vi "Can Rock Fall Down.vi"(0 "Position in Chamber to Check":i32, 1 "Chamber":u32[][](array[colorbox]), 2 "Rock":u32[][](array[colorbox])) -> (3 "Can Rock Fall Down ?":bool=TRUE)   [LabVIEW 2020, in "AoC 2022.lvlib"]
uses:
  AoC 2022.lvlib
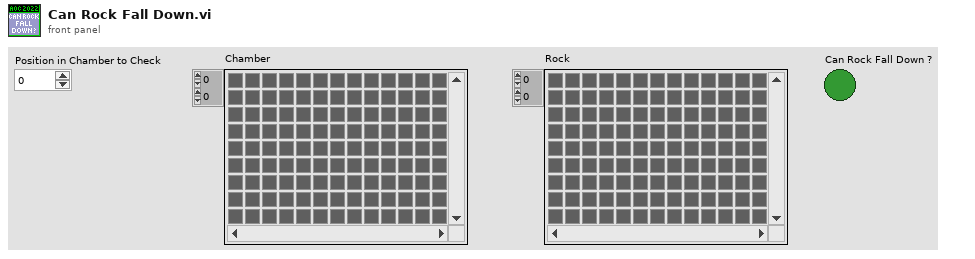
[diagram p1: front panel]
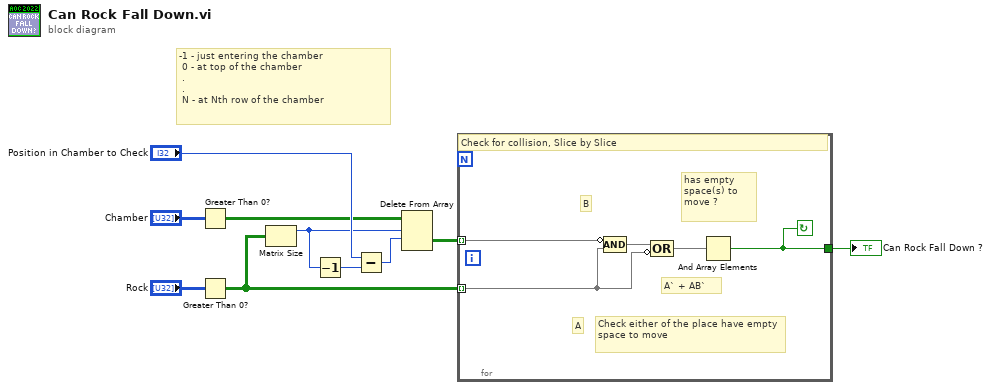
[diagram p0: block diagram]
diagram:
  # "-1 - just entering the chamber\n 0 - at top of the chamber\n .\n .\n N - at Nth row of the chamber"
  n1 = Greater Than 0?(x="Chamber") -> (x > 0?=w2:bool[][])
  n2 = Greater Than 0?(x="Rock") -> (x > 0?=w1:bool[][])
  n3 = Matrix Size(0:w1) -> (1:w5:i32)  [unwired: 1 out]
  n4 = Decrement(x=w5) -> (x-1=w3:i32)
  n5 = Subtract(x="Position in Chamber to Check", y=w3) -> (x-y=w4:i32)
  n6 = Delete From Array(array=w2, length=w5, index (row)=w4) -> (deleted portion=w7:bool[][])  [unwired: 1 in, 1 out]
  n7 = for {
    tunnel: [w12] -> w10
    tunnel: w1 -> [w13] mode=indexing
    tunnel: w7 -> [w11] mode=indexing
    stop <- w12 continue-if-true
    # "has empty space(s) to move ?"
    # "Check either of the place have empty space to move"
    # "B"
    # "A` + AB`"
    # "A"
    # "Check for collision, Slice by Slice"
    n8 = Compound Arithmetic op=AND(invert w11, w13) -> (w14:bool[])
    n9 = Compound Arithmetic op=OR(w14, invert w13) -> (w15:bool[])
    n10 = And Array Elements(Boolean array=w15) -> (logical AND=w12:bool)
  }
  "Can Rock Fall Down ?" <- w10
